vi "_Read.vi"(8 "error in (no error)":errorcluster, 11 "DAQ Analog in":refnum<class "DAQmx Analog.lvclass">) -> (0 "error out":errorcluster, 2 "4 Data Points":dbl[](array[numeric]), 3 "DAQ Analog out":refnum<class "DAQmx Analog.lvclass">)   [LabVIEW 2017, in "DAQmx Analog.lvclass"]
uses:
  DAQmx Analog.lvclass
  DAQmx Analog.lvclass/DAQmx Analog.ctl
  <vilib>/DAQmx/read.llb/DAQmx Read (Analog 1D DBL 1Chan NSamp).vi
  <vilib>/Analysis/baseanly.llb/Mean (DBL).vi
  <vilib>/DAQmx/miscellaneous.llb/DAQmx Fill In Error Info.vi
  <vilib>/Analysis/NI_AALBase.lvlib
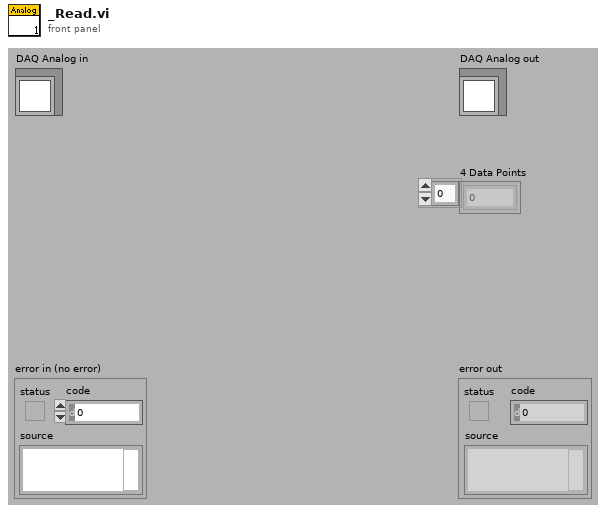
[diagram p1: front panel]
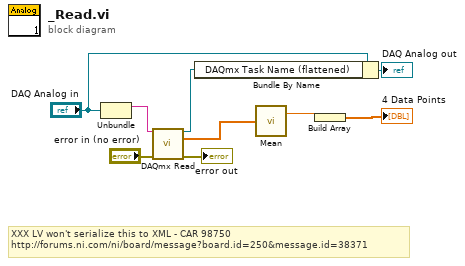
[diagram p0: block diagram]
diagram:
  # "XXX LV won't serialize this to XML - CAR 98750 \nhttp://forums.ni.com/ni/board/message?board.id=250&message.id=38371"
  n1 = Unbundle("DAQ Analog in") -> (w7:string)  [unwired: 1 out]
  n2 = call-poly <vilib>:"DAQmx Read.vi"("task/channels in"=w7, "error in"="error in (no error)") -> ("task out"=w3:refnum<k21>, "data"=w2:dbl[], "error out"=→"error out":errorcluster)  [unwired: 1 in, 10 out]
  n3 = Bundle By Name(cluster="DAQ Analog in", "DAQmx Task Name (flattened)"=w3) -> (→"DAQ Analog out":refnum<class "DAQmx Analog.lvclass">)
  n4 = call-poly <vilib>:"Mean.vi"("X"=w2) -> ("mean"=w1:dbl)  [unwired: 1 out]
  n5 = Build Array(w1) -> (→"4 Data Points":dbl[])
